vi "Main RT 2.vi"() -> ()   [LabVIEW 2015]
uses:
  <vilib>/RioEmbeddedCAN/RioEmbeddedCAN.llb/CANFrameControl.ctl
  Enum nastawy 2.ctl
  <vilib>/Platform/TimedLoop/XDataNode/timing_clust.ctl
  <vilib>/Platform/TimedLoop/XDataNode/nitl_modes.ctl
  <vilib>/Platform/TimedLoop/XDataNode/wakeup.ctl
  <vilib>/FPGAPlugInAG/sbRIO-9636/niLvFpga_Open_sbRIO-9636.vi
  <vilib>/rvi/interface/common/dynamic/niFpgaDynamicAddResources.vi
  <vilib>/FPGAPlugInAG/Dynamic/niLvFpga_Reset_Dynamic.vi
  <vilib>/FPGAPlugInAG/Dynamic/niLvFpga_Run_Dynamic.vi
  <vilib>/FPGAPlugInAG/Dynamic/niLvFpga_Close_Dynamic.vi
  <vilib>/platform/TimedLoop/XDataNode/XDataNode.xnode
  <vilib>/rvi/interface/nirviOpenFPGA/nirviOpenFPGA.xnode
  FPGA Bitfiles/Raptorv2_FPGATarget_FPGAMain_nw1CBh-YlYM.lvbitx
  FPGA/Main FPGA.vi
  <vilib>/rvi/interface/nirviMethod/nirviMethod.xnode
  <vilib>/rvi/interface/nirviCloseFPGA/nirviCloseFPGA.xnode
  <vilib>/Platform/TimedLoop/XDataNode/XDNodeRunTimeDep.lvlib
  <vilib>/robotics/Protocols/NMEA/NMEA API.lvlib
  <vilib>/Instr/_visa.llb/VISA Configure Serial Port (Instr).vi
  <resource>/objmgr/RioEmbeddedCANInterface.rc
panel:
  out "specific error cleared?":bool
  in  "Boolean":bool
  in  "ramki jazdy 2":T1[](array[typedef]) {"type" items=["CAN Data", "CAN Remote"]; "identifier" format="%.0x"}
  out "Numeric":i32
  out "# pending insert":i32
  out "# pending remove":i32
  out "# elements in queue":i32
  out "current time":timestamp
  out "Delay":dbl
  out "Odebrane wiadomości z PC":dbl
  out "CAN frame":T1 {"type" items=["CAN Data", "CAN Remote"]; "identifier" format="%.0x"}
  out "Przestarzała data":bool caption="Time has Elapsed"
  out "longitude (deg) 2":dbl format="%#_8g"
  out "latitude (deg) 2":dbl format="%#_8g"
  in  "VISA resource name":refnum<visa-resource-name>="ASRL1::INSTR"
  out "longitude (deg)":i64
  out "latitude (deg)":i64
  out "GPS data":T2 {"oldest read timestamp" format="%^<%.3X\n%x>T"; "latitude (deg)" format="%#_10g"; "longitude (deg)" format="%#_10g"}
  out "wyczyszczona":bool=TRUE
  in  "Wyczyśćkolejke":bool
  in  "stop wysylanie":bool
  in  "odczyt CAN-a":bool=TRUE
  out "ilosc mesagy READ CAN":dbl
  in  "Pokaz odczytany CAN":bool=TRUE
  out "CAN Frames":string[][](table) caption="Frames"
  in  "stop odczyt can":bool
  in  "Hexadecimal?":bool
  in  "stop zapis can":bool
  out "new data":bool
  out "ramki jazdy":T1[](array[typedef]) {"type" items=["CAN Data", "CAN Remote"]; "identifier" format="%.0x"}
  in  "odbior udp":bool
  out "ramki konf":T1 {"type" items=["CAN Data", "CAN Remote"]; "identifier" format="%.0x"}
  in  "Number of Frames to Display":i32=5
  in  "receive queue size":u32=500
  in  "baud rate":u32=500000
  in  "interface index":u32
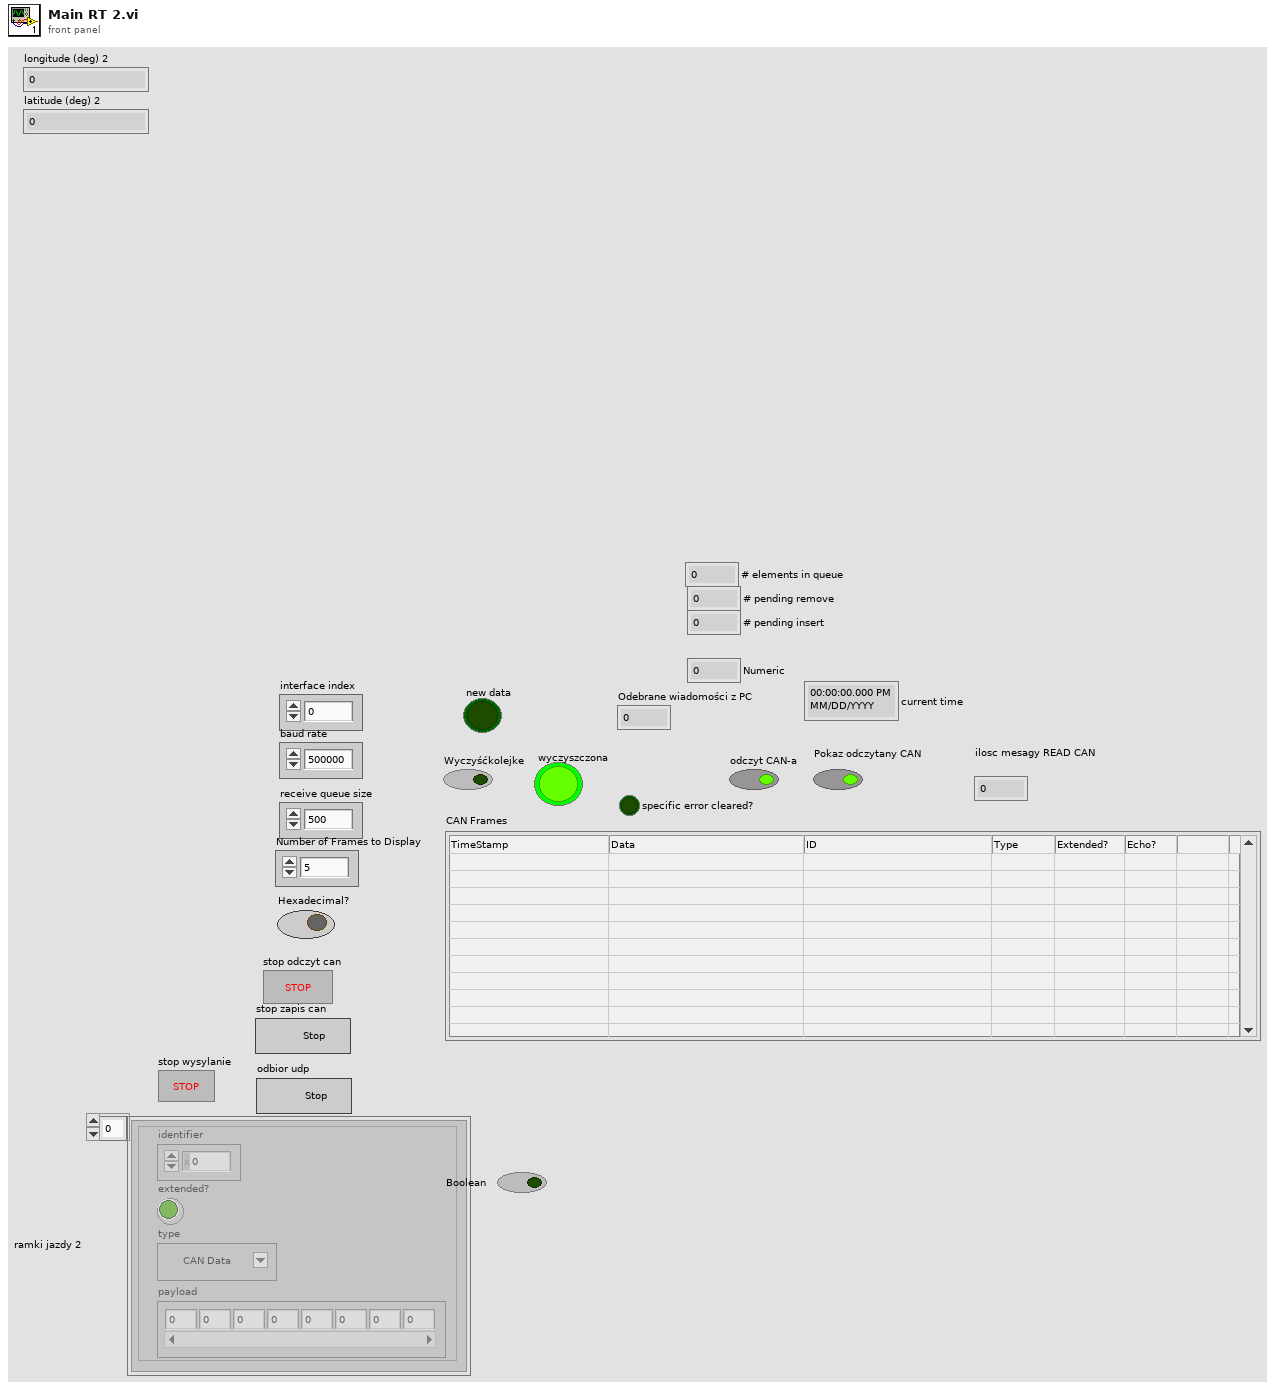
[diagram p1: front panel]
types:
  T1 = typedef "CANFrameControl.ctl" = cluster{"identifier":u32, "extended?":bool, "type":u8, "payload":u8[]}
  T2 = cluster{"oldest read timestamp":timestamp, "latitude (deg)":dbl, "longitude (deg)":dbl, "ground speed (knots)":dbl, "true track angle (deg)":dbl, "altitude above mean sea level (m)":dbl}
  T3 = typedef "Enum nastawy 2.ctl" = enum16{"STOP", "PRZOD P", "SRODEK P", "TYL P", "PRZOD L", "SRODEK L", "TYL L"}
  T4 = typedef "XDNodeRunTimeDep.lvlib/timing_clust.ctl" = cluster{"Expected End [f-1]":u64, "Actual End [f-1]":u64, "Finished Late? [f-1]":bool, "Expected End [i-1]":u64, "Actual End [i-1]":u64, "Finished Late? [i-1]":bool, "Expected Start [i]":u64, "Actual Start [i]":u64, "Expected Start [f]":u64, "Actual Start [f]":u64, "Source Name":string, "Structure Name":string, "Period":i64, "Deadline":i64, "Offset":i64, "Start":i64, "Priority":i32, "Timeout":i32, "Mode":T5, "Wakeup Reason":T6, "Error":errorcluster, "Source Type":string, "Secondary Source Type":string, "Global End Time":u64, "Global Start Time":u64, "Frame Duration":u64, "Iteration Duration":u64, "Assigned CPU":i32, "I/O Scan Engine Mode":u32}
  T5 = typedef "XDNodeRunTimeDep.lvlib/nitl_modes.ctl" = enum32{"No Change", "Process missed periods, maintain original phase", "Discard missed periods, maintain original phase", "Process missed periods, ignore original phase", "Discard missed periods, ignore original phase"}
  T6 = typedef "XDNodeRunTimeDep.lvlib/wakeup.ctl" = enum32{"Normal", "Aborted", "Asynchronous wakeup", "Timing source error", "Timed loop error", "Timeout"}
  T7 = cluster{"type":string, "Cluster":cluster{"date/time string":string, "array of cans":T1[]}, "bool":bool}
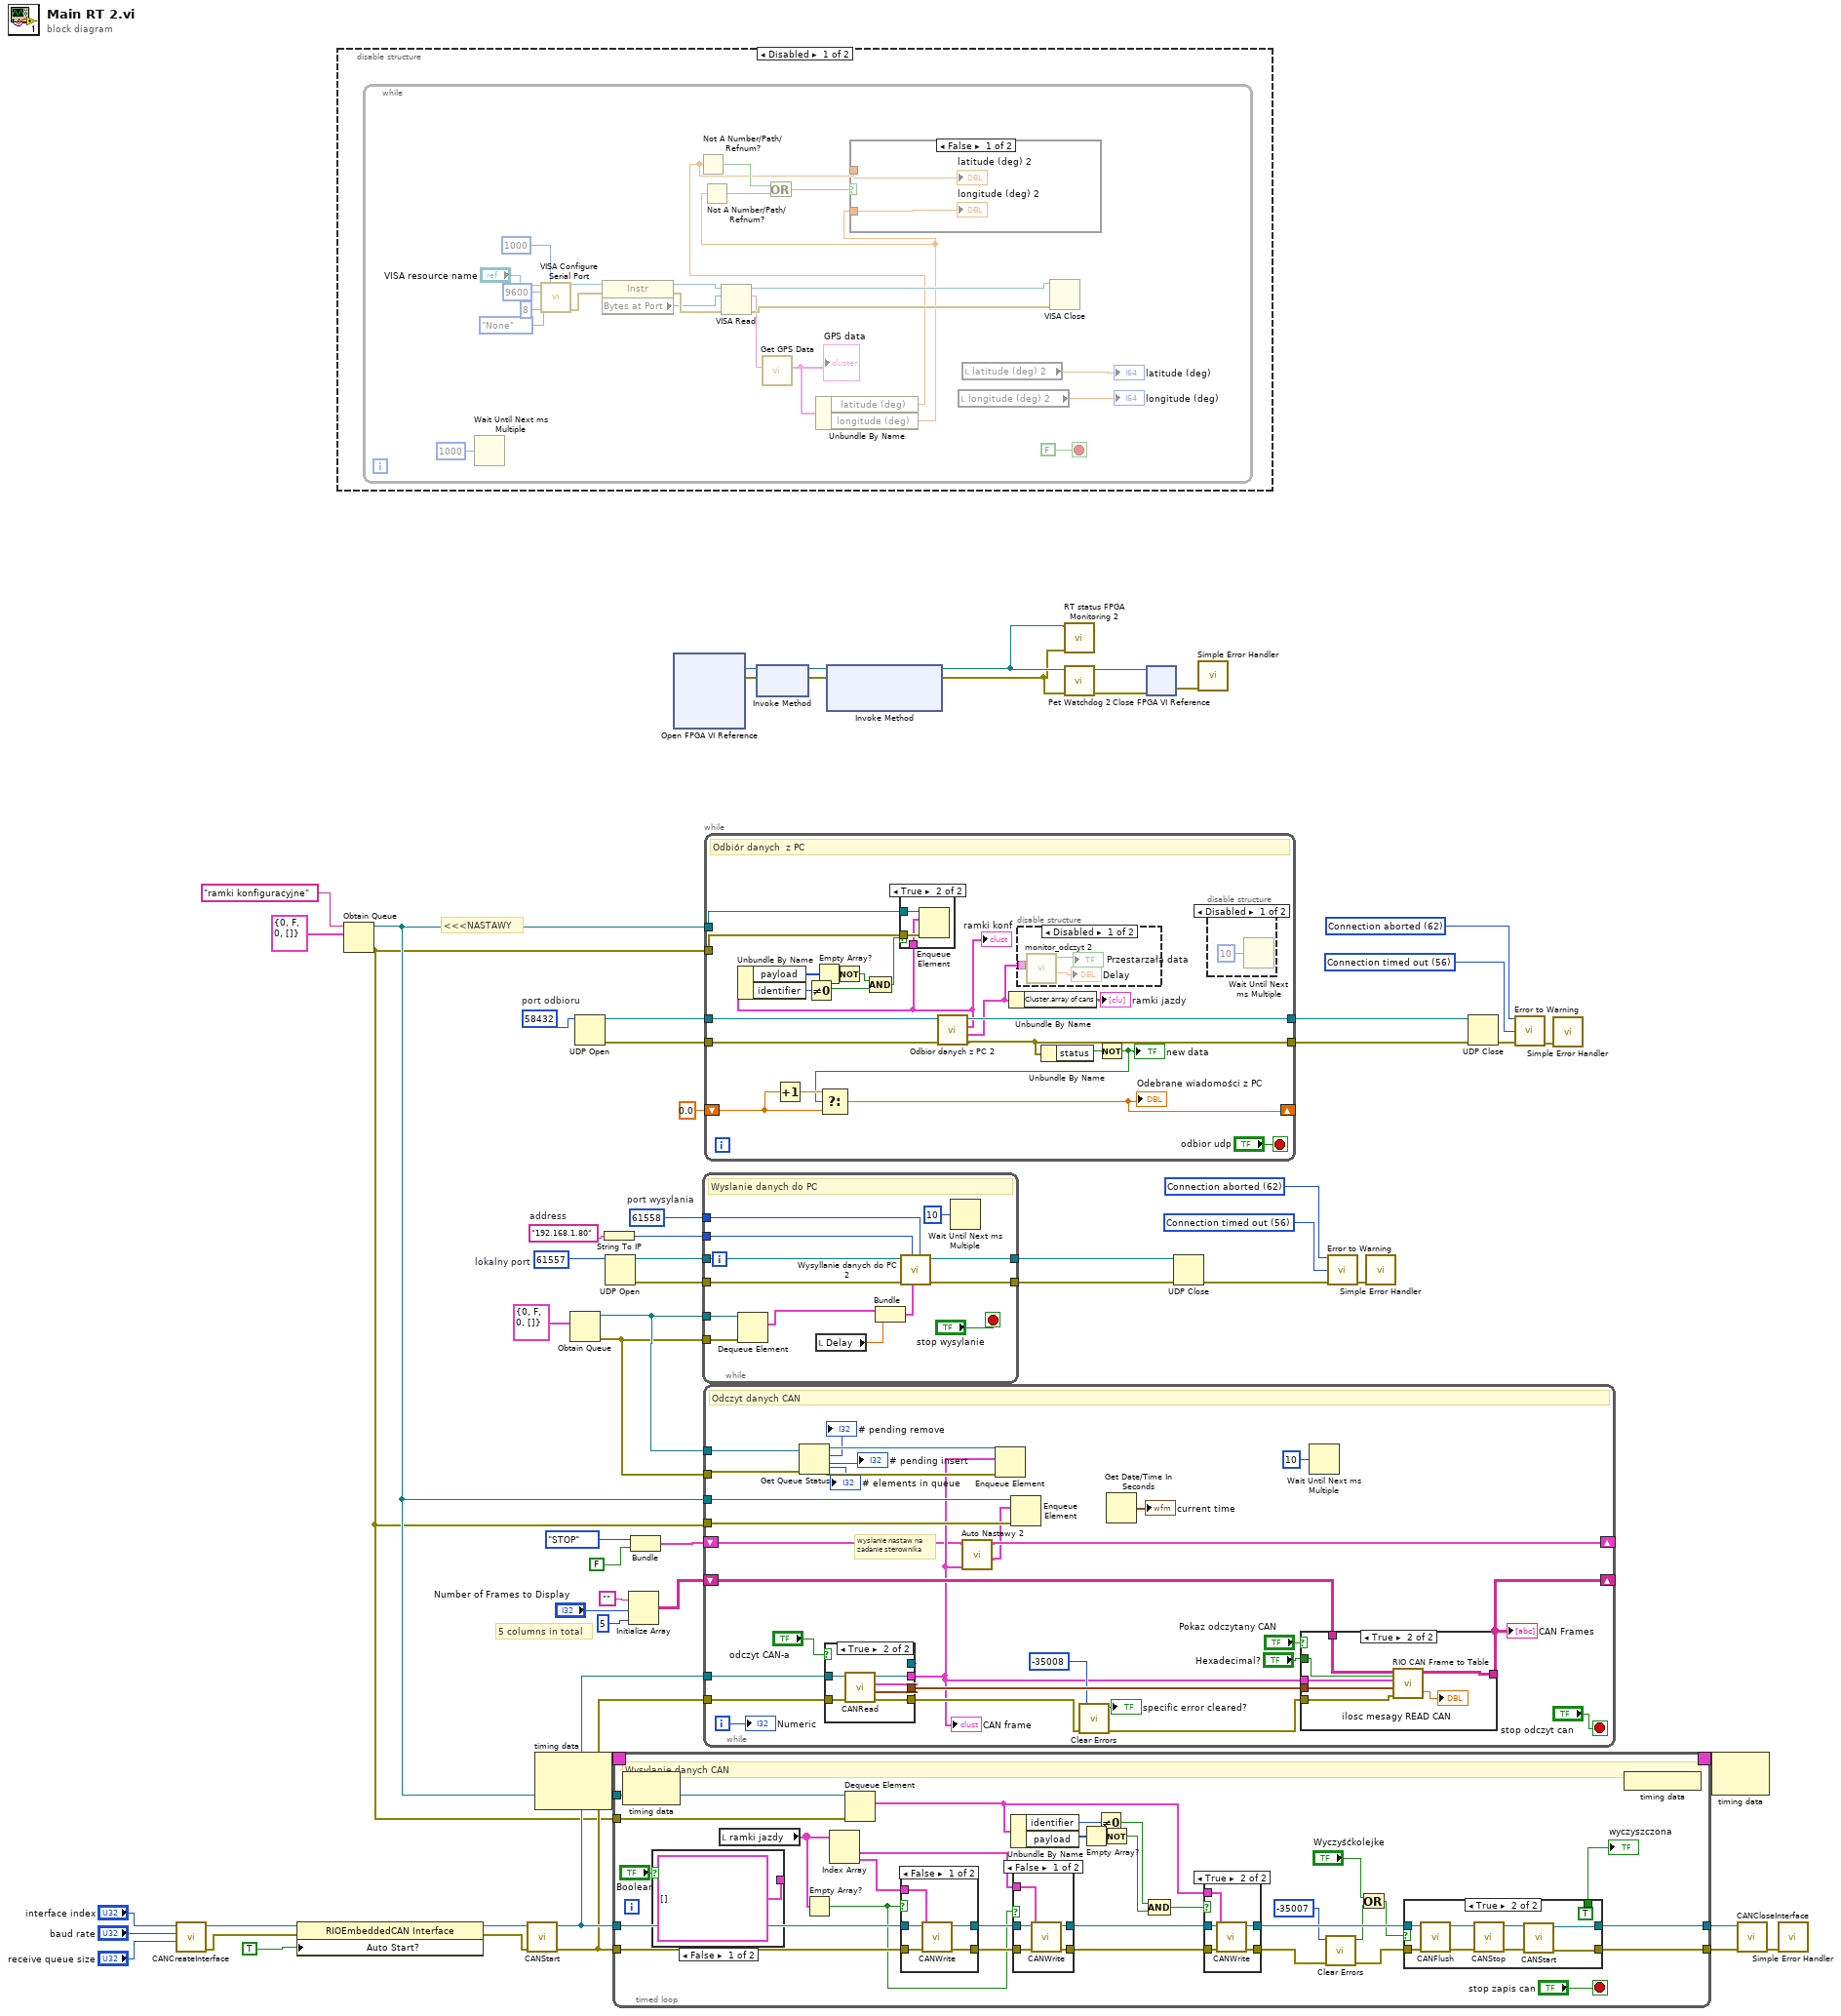
[diagram p0: block diagram]
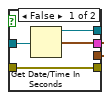
[diagram p3: hidden frame]
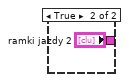
[diagram p9: hidden frame]
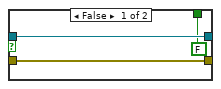
[diagram p10: hidden frame]
diagram:
  w22 = u16 58432  # port odbioru
  w26 = 56 items=["No Error", "Argument Error", "Memory Full", "Out of Zone", "End of File", "File Already Open", "Generic File IO Error", "File Not Found", "File Permission Error", "Disk Full", "Duplicate Path", "Too Many Files Open", "Not Enabled", "Resource File Not Found", "Cannot Add Resource", "Resource Not Found", "Image Not Found", "Image Memory Error", "Pen Does Not Exist", "Config Bad Type", "Config Token Not Found", "Config Parse Error", "Config Memory Error", "Bad External Code Format", "Bad External Code Offset", "External Code Not Present", "Null Window", "Destroy Window Mixup", "Null Menu", "Print Aborted", "Bad Print Record", "Print Driver Error", "Windows Error During Print", "Memory Error During Print", "Print Dialog Error", "Generic Print Error", "Invalid Device Refnum", "Device Not Found", "Device Parameter Error", "Device Unit Error", "Can't Open Device", "Device Call Aborted", "Generic Error", "Cancelled By User", "Object ID Too Low", "Object ID Too High", "Object Not In Heap", "Unknown Heap", "Bad DefProc ID", "DefProc Not In Table", "Message Out Of Range", "Null Method", "Unknown Message", "Manager Call Not Supported", "Bad address", "Connection In progress", "Connection timed out", "Connection is already in progress", "Network attribute not supported", "Network error", "Address in use", "System out of memory", "Connection aborted", "Connection refused", "Connection is not connected", "Connection is already connected", "Connection closed", "Initialize error (interapplication manager)", "Bad occurrence", "Wait on unbound occurrence handler", "Occurrence queue overflow", "Bad path", "Semaphore not signaled", "Unrecognized type (interapplication manager)"] ("3rd Error to Convert")
  w25 = 62 items=["No Error", "Argument Error", "Memory Full", "Out of Zone", "End of File", "File Already Open", "Generic File IO Error", "File Not Found", "File Permission Error", "Disk Full", "Duplicate Path", "Too Many Files Open", "Not Enabled", "Resource File Not Found", "Cannot Add Resource", "Resource Not Found", "Image Not Found", "Image Memory Error", "Pen Does Not Exist", "Config Bad Type", "Config Token Not Found", "Config Parse Error", "Config Memory Error", "Bad External Code Format", "Bad External Code Offset", "External Code Not Present", "Null Window", "Destroy Window Mixup", "Null Menu", "Print Aborted", "Bad Print Record", "Print Driver Error", "Windows Error During Print", "Memory Error During Print", "Print Dialog Error", "Generic Print Error", "Invalid Device Refnum", "Device Not Found", "Device Parameter Error", "Device Unit Error", "Can't Open Device", "Device Call Aborted", "Generic Error", "Cancelled By User", "Object ID Too Low", "Object ID Too High", "Object Not In Heap", "Unknown Heap", "Bad DefProc ID", "DefProc Not In Table", "Message Out Of Range", "Null Method", "Unknown Message", "Manager Call Not Supported", "Bad address", "Connection In progress", "Connection timed out", "Connection is already in progress", "Network attribute not supported", "Network error", "Address in use", "System out of memory", "Connection aborted", "Connection refused", "Connection is not connected", "Connection is already connected", "Connection closed", "Initialize error (interapplication manager)", "Bad occurrence", "Wait on unbound occurrence handler", "Occurrence queue overflow", "Bad path", "Semaphore not signaled", "Unrecognized type (interapplication manager)"] ("1st Error to Convert")
  w35 = u16 61557  # lokalny port
  w33 = u16 61558  # port wysylania
  w34 = "192.168.1.80"  # address
  w37 = 56 items=["No Error", "Argument Error", "Memory Full", "Out of Zone", "End of File", "File Already Open", "Generic File IO Error", "File Not Found", "File Permission Error", "Disk Full", "Duplicate Path", "Too Many Files Open", "Not Enabled", "Resource File Not Found", "Cannot Add Resource", "Resource Not Found", "Image Not Found", "Image Memory Error", "Pen Does Not Exist", "Config Bad Type", "Config Token Not Found", "Config Parse Error", "Config Memory Error", "Bad External Code Format", "Bad External Code Offset", "External Code Not Present", "Null Window", "Destroy Window Mixup", "Null Menu", "Print Aborted", "Bad Print Record", "Print Driver Error", "Windows Error During Print", "Memory Error During Print", "Print Dialog Error", "Generic Print Error", "Invalid Device Refnum", "Device Not Found", "Device Parameter Error", "Device Unit Error", "Can't Open Device", "Device Call Aborted", "Generic Error", "Cancelled By User", "Object ID Too Low", "Object ID Too High", "Object Not In Heap", "Unknown Heap", "Bad DefProc ID", "DefProc Not In Table", "Message Out Of Range", "Null Method", "Unknown Message", "Manager Call Not Supported", "Bad address", "Connection In progress", "Connection timed out", "Connection is already in progress", "Network attribute not supported", "Network error", "Address in use", "System out of memory", "Connection aborted", "Connection refused", "Connection is not connected", "Connection is already connected", "Connection closed", "Initialize error (interapplication manager)", "Bad occurrence", "Wait on unbound occurrence handler", "Occurrence queue overflow", "Bad path", "Semaphore not signaled", "Unrecognized type (interapplication manager)"] ("3rd Error to Convert")
  w18 = 62 items=["No Error", "Argument Error", "Memory Full", "Out of Zone", "End of File", "File Already Open", "Generic File IO Error", "File Not Found", "File Permission Error", "Disk Full", "Duplicate Path", "Too Many Files Open", "Not Enabled", "Resource File Not Found", "Cannot Add Resource", "Resource Not Found", "Image Not Found", "Image Memory Error", "Pen Does Not Exist", "Config Bad Type", "Config Token Not Found", "Config Parse Error", "Config Memory Error", "Bad External Code Format", "Bad External Code Offset", "External Code Not Present", "Null Window", "Destroy Window Mixup", "Null Menu", "Print Aborted", "Bad Print Record", "Print Driver Error", "Windows Error During Print", "Memory Error During Print", "Print Dialog Error", "Generic Print Error", "Invalid Device Refnum", "Device Not Found", "Device Parameter Error", "Device Unit Error", "Can't Open Device", "Device Call Aborted", "Generic Error", "Cancelled By User", "Object ID Too Low", "Object ID Too High", "Object Not In Heap", "Unknown Heap", "Bad DefProc ID", "DefProc Not In Table", "Message Out Of Range", "Null Method", "Unknown Message", "Manager Call Not Supported", "Bad address", "Connection In progress", "Connection timed out", "Connection is already in progress", "Network attribute not supported", "Network error", "Address in use", "System out of memory", "Connection aborted", "Connection refused", "Connection is not connected", "Connection is already connected", "Connection closed", "Initialize error (interapplication manager)", "Bad occurrence", "Wait on unbound occurrence handler", "Occurrence queue overflow", "Bad path", "Semaphore not signaled", "Unrecognized type (interapplication manager)"] ("1st Error to Convert")
  # "<<<NASTAWY"
  # "5 columns in total"
  n1 = call <vilib>:"CANCreateInterface.vi"("receive queue size (5)"="receive queue size", "baud rate (125000 bps)"="baud rate", "interface index"="interface index") -> ("error out"=w7:errorcluster, "interface object out"=w10:refnum<k20>)  [unwired: 7 in]
  n2 = property class="RIOEmbeddedCAN Interface"(reference=w10, error in=w7, "Auto Start?"=TRUE) -> (reference out=w8:refnum<k20>, error out=w6:errorcluster)
  n3 = disable-structure shown="Disabled" {
    frame Disabled {
      n4 = while {
        stop <- FALSE stop-if-true
        n5 = Wait Until Next ms Multiple(millisecond multiple=u32 1000) -> ()  [unwired: 1 out]
        n6 = call-poly "VISA Configure Serial Port"("VISA resource name"="VISA resource name", "timeout (10sec)"=u32 1000, "baud rate (9600)"=u32 9600, "data bits (8)"=u16 8, "parity (0:none)"=enum16{"None", "Odd", "Even", "Mark", "Space"}."None") -> ("VISA resource name out"=w80:refnum<visa-resource-name>, "error out"=w79:errorcluster)  [unwired: 9 in]
        n7 = property class="Instr"(reference=w80, error in=w79) -> (reference out=w81:refnum<visa-resource-name>, error out=w78:errorcluster, "Bytes at Port"=w74:u32)
        n8 = VISA Read(VISA resource name=w81, byte count=w74, error in (no error)=w78) -> (VISA resource name out=w82:refnum<visa-resource-name>, read buffer=w76:string, error out=w77:errorcluster)  [unwired: 1 out]
        n9 = call <vilib>:"Get GPS Data.vi"("sensor data"=w76) -> ("GPS data"=w75:T2)  [unwired: 8 in, 2 out]
        "GPS data" <- w75
        n10 = Unbundle By Name(w75) -> ("latitude (deg)"=w64:dbl, "longitude (deg)"=w62:dbl)
        n11 = Not A Number/Path/Refnum?(number/path/refnum=w64) -> (NaN/Path/Refnum?=w67:bool)
        n12 = Not A Number/Path/Refnum?(number/path/refnum=w62) -> (NaN/Path/Refnum?=w66:bool)
        n13 = Or(x=w67, y=w66) -> (x .or. y?=w65:bool)
        n14 = case shown="False" w65 {
          tunnel: w62 -> [w85 _]
          tunnel: w64 -> [w84 _]
          frame False {
            "longitude (deg) 2" <- w85
            "latitude (deg) 2" <- w84
          }
          frame True {
          }
        }
        n15 = local read "longitude (deg) 2"() -> (→"longitude (deg)":dbl)
        n16 = local read "latitude (deg) 2"() -> (→"latitude (deg)":dbl)
        n17 = VISA Close(VISA resource name=w82, error in (no error)=w77) -> ()  [unwired: 1 out]
      }
    }
    frame Enabled {
    }
  }
  n18 = Obtain Queue(name (unnamed)="ramki konfiguracyjne", element data type=T1 {"identifier"=0, "extended?"=FALSE, "type"=0, "payload"=[]} ("ramki konf")) -> (queue out=w15:refnum<queue>, error out=w14:errorcluster)  [unwired: 3 in, 1 out]
  n19 = call <vilib>:"CANStart.vi"("error in (no error)"=w6, "interface object in"=w8) -> ("error out"=w47:errorcluster, "interface object out"=w48:refnum<k20>)  [unwired: 8 in]
  n20 = node-c288() -> (w60:T4)  [unwired: 2 in]
  n21 = Obtain Queue(element data type=T1 {"identifier"=0, "extended?"=FALSE, "type"=0, "payload"=[]} ("CAN frame")) -> (queue out=w12:refnum<queue>, error out=w11:errorcluster)  [unwired: 4 in, 1 out]
  n22 = UDP Open(11:w22) -> (port=w39:refnum<k16>, 0:w40:errorcluster)  [unwired: 4 in, 1 out]
  n23 = String To IP(1:w34) -> (0:w32:u32)
  n24 = UDP Open(11:w35) -> (port=w31:refnum<k16>, 0:w30:errorcluster)  [unwired: 4 in, 1 out]
  n25 = timed-loop "Timed Loop" {
    tunnel: w48 -> [w103]
    tunnel: w47 -> [w102]
    tunnel: [w101] -> w51
    tunnel: [w100] -> w50
    timing: w60 -> [_]
    timing-out: [_] -> w59
    tunnel: w15 -> [w91]
    tunnel: w14 -> [w90]
    stop <- "stop zapis can" stop-if-true
    # "Wysylanie danych CAN"
    n26 = node-c288() -> ()  [unwired: 1 in, 1 out]
    n27 = case shown="False" "Boolean" {
      tunnel: [T1[] [] ("ramki jazdy 2") "ramki jazdy 2"] -> _
      frame False {
      }
      frame True {
      }
    }
    n28 = local read "ramki jazdy"() -> (w86:T1[])
    n29 = Empty Array?(array=w86) -> (empty?=w88:bool)
    n30 = Index Array(array=w86) -> (element #1=w114:T1, element #2=w113:T1)  [unwired: 2 in]
    n31 = Dequeue Element(queue=w91, error in (no error)=w90) -> (element=w89:T1)  [unwired: 1 in, 3 out]
    n32 = case shown="False" w88 {
      tunnel: w103 -> [w151 w152]
      tunnel: w102 -> [w150 w153]
      tunnel: [w148 w152] -> w115
      tunnel: [w147 w153] -> w116
      tunnel: w113 -> [w149 _]
      frame False {
        n33 = call <vilib>:"CANWrite.vi"("error in (no error)"=w150, "CAN frame"=w149, "interface object in"=w151) -> ("error out"=w147:errorcluster, "interface object out"=w148:refnum<k20>)  [unwired: 7 in]
      }
      frame True {
      }
    }
    n34 = Unbundle By Name(w89) -> ("identifier"=w109:u32, "payload"=w110:u8[])
    n35 = case shown="False" w88 {
      tunnel: w116 -> [w144 w146]
      tunnel: [w142 w145] -> w112
      tunnel: [w141 w146] -> w111
      tunnel: w115 -> [w143 w145]
      tunnel: w114 -> [w140 _]
      frame False {
        n36 = call <vilib>:"CANWrite.vi"("error in (no error)"=w144, "CAN frame"=w140, "interface object in"=w143) -> ("error out"=w141:errorcluster, "interface object out"=w142:refnum<k20>)  [unwired: 7 in]
      }
      frame True {
      }
    }
    n37 = Empty Array?(array=w110) -> (empty?=w106:bool)
    n38 = Not Equal To 0?(x=w109) -> (x != 0?=w107:bool)
    n39 = Not(x=w106) -> (.not. x?=w105:bool)
    n40 = Compound Arithmetic op=AND(w107, w105) -> (w108:bool)
    n41 = case shown="True" w108 {
      tunnel: w111 -> [w132 w137]
      tunnel: [w131 w134] -> w99
      tunnel: [w132 w133] -> w104
      tunnel: w112 -> [w131 w136]
      tunnel: w89 -> [_ w135]
      frame False {
      }
      frame True {
        n42 = call <vilib>:"CANWrite.vi"("error in (no error)"=w137, "CAN frame"=w135, "interface object in"=w136) -> ("error out"=w133:errorcluster, "interface object out"=w134:refnum<k20>)  [unwired: 7 in]
      }
    }
    n43 = call <vilib>:"Clear Errors.vi"("error in (no error)"=w104, "specific error code to clear (0: all)"=-35007) -> ("error out"=w96:errorcluster, "specific error cleared?"=w94:bool)  [unwired: 4 in]
    n44 = Or(x="Wyczyśćkolejke", y=w94) -> (x .or. y?=w95:bool)
    n45 = case shown="True" w95 {
      tunnel: [w121 w123] -> w101
      tunnel: [w120 w122] -> w100
      tunnel: w99 -> [w121 w130]
      tunnel: w96 -> [w120 w129]
      tunnel: [FALSE TRUE] -> w92
      frame False {
      }
      frame True {
        n46 = call <vilib>:"CANFlush.vi"("error in (no error)"=w129, "interface object in"=w130) -> ("error out"=w126:errorcluster, "interface object out"=w127:refnum<k20>)  [unwired: 8 in]
        n47 = call <vilib>:"CANStop.vi"("error in (no error)"=w126, "interface object in"=w127) -> ("error out"=w125:errorcluster, "interface object out"=w124:refnum<k20>)  [unwired: 8 in]
        n48 = call <vilib>:"CANStart.vi"("error in (no error)"=w125, "interface object in"=w124) -> ("error out"=w122:errorcluster, "interface object out"=w123:refnum<k20>)  [unwired: 8 in]
      }
    }
    "wyczyszczona" <- w92
    n49 = node-c288() -> ()  [unwired: 1 out]
  }
  n50 = Initialize Array("" ("Empty String Constant"), "Number of Frames to Display", 5 ("dimension size")) -> (w49:string[][])
  n51 = Bundle("Enum"=Enum_nastawy_2."STOP", FALSE) -> (w17:cluster{"Enum":T3, bool})  [unwired: 1 in]
  n52 = xnode "Open FPGA VI Reference"() -> ("FPGA VI Reference Out"=w43:refnum<k20>, "error out"=w44:errorcluster)  [unwired: 2 in]
  n53 = while {
    tunnel: w33 -> [w158]
    tunnel: w32 -> [w159]
    tunnel: w31 -> [w160]
    tunnel: w30 -> [w155]
    tunnel: [w157] -> w29
    tunnel: [w156] -> w28
    tunnel: w12 -> [w163]
    tunnel: w11 -> [w162]
    stop <- "stop wysylanie" stop-if-true
    # "Wyslanie danych do PC"
    n54 = Dequeue Element(queue=w163, error in (no error)=w162) -> (element=w161:T1)  [unwired: 1 in, 3 out]
    n55 = local read "Delay"() -> (w164:dbl)
    n56 = Bundle("CAN frame"=w161, "Delay"=w164) -> (w154:cluster{"CAN frame":T1, "Delay":dbl})  [unwired: 1 in]
    n57 = call "Wysyllanie danych do PC  2.vi"("remote port"=w158, "output cluster"=w154, "adres"=w159, "error in (no error)"=w155, "UDP Network Connection in"=w160) -> ("error out"=w156:errorcluster, "UDP Network Connection out"=w157:refnum<k16>)  [unwired: 5 in]
    n58 = Wait Until Next ms Multiple(millisecond multiple=u32 10) -> ()  [unwired: 1 out]
  }
  n59 = while "Timed Loop" {
    shift-right: [w188] -> _
    shift-left: w49 -> [w189]
    tunnel: w48 -> [w195]
    tunnel: w47 -> [w194]
    shift-right: [w168] -> _
    shift-left: w17 -> [w169]
    tunnel: w15 -> [w193]
    tunnel: w14 -> [w192]
    tunnel: w12 -> [w191]
    tunnel: w11 -> [w190]
    i -> [w177]
    stop <- "stop odczyt can" stop-if-true
    # "wyslanie nastaw na \nzadanie sterownika"
    # "Odczyt danych CAN"
    n60 = Get Queue Status(queue=w191, error in (no error)=w190) -> (queue out=w182:refnum<queue>, # pending remove=→"# pending remove":i32, # pending insert=→"# pending insert":i32, error out=w181:errorcluster, # elements in queue=→"# elements in queue":i32)  [unwired: 1 in, 3 out]
    n61 = case shown="True" "odczyt CAN-a" {
      tunnel: w195 -> [w205 w212]
      tunnel: w194 -> [w206 w211]
      tunnel: [w204 w210] -> w186
      tunnel: [w206 w209] -> w174
      tunnel: [_ w207] -> w170
      tunnel: [w205 w208] -> _
      frame False {
        n62 = Get Date/Time In Seconds() -> (seconds since 1Jan1904=w204:timestamp)
      }
      frame True {
        n63 = call <vilib>:"CANRead.vi"("error in (no error)"=w211, "interface object in"=w212) -> ("error out"=w209:errorcluster, "timestamp"=w210:timestamp, "CAN frame"=w207:T1, "interface object out"=w208:refnum<k20>)  [unwired: 6 in]
      }
    }
    "CAN frame" <- w170
    n64 = call "Auto Nastawy 2.vi"("CAN ramki in"=w170, "Auto N in"=w169) -> ("CAN konifguracyjny"=w167:T1, "Auto N out"=w168:cluster{"Enum":T3, bool})  [unwired: 8 in]
    n65 = Enqueue Element(queue=w182, element=w170, error in (no error)=w181) -> ()  [unwired: 1 in, 3 out]
    n66 = Enqueue Element(queue=w193, element=w167, error in (no error)=w192) -> ()  [unwired: 1 in, 3 out]
    n67 = call <vilib>:"Clear Errors.vi"("error in (no error)"=w174, "specific error code to clear (0: all)"=-35008) -> ("error out"=w173:errorcluster, "specific error cleared?"=→"specific error cleared?":bool)  [unwired: 4 in]
    n68 = Get Date/Time In Seconds() -> (seconds since 1Jan1904=→"current time":timestamp)
    n69 = case shown="True" "Pokaz odczytany CAN" {
      tunnel: [w196 w203] -> w188
      tunnel: w189 -> [w196 w201]
      tunnel: w186 -> [_ w200]
      tunnel: w170 -> [_ w199]
      tunnel: w173 -> [_ w198]
      tunnel: "Hexadecimal?" -> [_ w197]
      frame False {
      }
      frame True {
        n70 = call "RIO CAN Frame to Table.vi"("Hexadecimal?"=w197, "error in (no error)"=w198, "timestamp"=w200, "CAN frame"=w199, "Old CAN Frames"=w201) -> ("New CAN Frames"=w203:string[][], "Ilość wiadomości CAN odebranych"=→"ilosc mesagy READ CAN":dbl)  [unwired: 5 in]
      }
    }
    "CAN Frames" <- w188
    n71 = Wait Until Next ms Multiple(millisecond multiple=u32 10) -> ()  [unwired: 1 out]
    "Numeric" <- w177
  }
  n72 = while {
    tunnel: w39 -> [w218]
    tunnel: w40 -> [w217]
    tunnel: [w216] -> w41
    tunnel: [w215] -> w23
    tunnel: w15 -> [w231]
    tunnel: w14 -> [w230]
    shift-right: [w223] -> _
    shift-left: 0.0 -> [w222]
    stop <- "odbior udp" stop-if-true
    # "Odbiór danych  z PC"
    n73 = Increment(x=w222) -> (x+1=w224:dbl)
    n74 = call "Odbior danych z PC 2.vi"("error in (no error)"=w217, "connection ID"=w218) -> ("error out"=w216:errorcluster, "output cluster"=w213:T7, "konf"=w214:T1, "connection ID out"=w215:refnum<k16>)  [unwired: 6 in]
    "ramki konf" <- w214
    n75 = Unbundle By Name(w214) -> ("payload"=w228:u8[], "identifier"=w229:u32)
    n76 = Not Equal To 0?(x=w229) -> (x != 0?=w226:bool)
    n77 = Empty Array?(array=w228) -> (empty?=w220:bool)
    n78 = Not(x=w220) -> (.not. x?=w227:bool)
    n79 = Compound Arithmetic op=AND(w227, w226) -> (w225:bool)
    n80 = case shown="True" w225 {
      tunnel: w231 -> [_ w239]
      tunnel: w230 -> [_ w238]
      tunnel: w214 -> [_ w237]
      frame False {
      }
      frame True {
        n81 = Enqueue Element(queue=w239, element=w237, error in (no error)=w238) -> ()  [unwired: 1 in, 3 out]
      }
    }
    n82 = Unbundle By Name(w213) -> ("Cluster.array of cans"=→"ramki jazdy":T1[])
    n83 = disable-structure shown="Disabled" {
      disable-tunnel: w213 -> [w234 _]
      frame Disabled {
        n84 = call "monitor_odczyt 2.vi"("output cluster"=w234) -> ("Delay"=→"Delay":dbl, "Przestarzała data"=→"Przestarzała data":bool)  [unwired: 8 in, 1 out]
      }
      frame Enabled {
      }
    }
    n85 = Unbundle By Name(w216) -> ("status"=w232:bool)
    n86 = Not(x=w232) -> (.not. x?=w221:bool)
    "new data" <- w221
    n87 = Select(t=w224, s=w221, f=w222) -> (s? t:f=w223:dbl)
    "Odebrane wiadomości z PC" <- w223
    n88 = disable-structure shown="Disabled" {
      frame Disabled {
        n89 = Wait Until Next ms Multiple(millisecond multiple=u32 10) -> ()  [unwired: 1 out]
      }
      frame Enabled {
      }
    }
  }
  n90 = xnode "Invoke Method"("FPGA VI Reference In"=w43, "error in"=w44) -> ("FPGA VI Reference Out"=w45:refnum<k20>, "error out"=w46:errorcluster)
  n91 = xnode "Invoke Method"("FPGA VI Reference In"=w45, "error in"=w46) -> ("FPGA VI Reference Out"=w4:refnum<k20>, "error out"=w1:errorcluster)  [unwired: 1 in]
  n92 = call "RT status FPGA Monitoring 2.vi"("error in (no error)"=w1, "FPGA VI Reference Out 2"=w4) -> ()  [unwired: 10 in]
  n93 = call "Pet Watchdog 2.vi"("error in (no error)"=w1, "FPGA VI Reference Out"=w4) -> ("error out"=w2:errorcluster, "FPGA VI Reference Out 2"=w3:refnum<k20>)  [unwired: 8 in]
  n94 = xnode "Close FPGA VI Reference"("FPGA VI Reference In"=w3, "error in"=w2) -> ("error out"=w42:errorcluster)
  n95 = UDP Close(connection ID=w29, 8:w28) -> (error out=w38:errorcluster)  [unwired: 1 out]
  n96 = call <vilib>:"Simple Error Handler.vi"("error in (no error)"=w42) -> ()  [unwired: 1 in, 8 out]
  n97 = call <vilib>:"Error to Warning.vi"("1st Error to Convert"=w18, "3rd Error to Convert"=w37, "error in"=w38) -> ("warning out"=w36:errorcluster)  [unwired: 3 in, 9 out]
  n98 = call <vilib>:"Simple Error Handler.vi"("error in (no error)"=w36) -> ()  [unwired: 1 in, 8 out]
  n99 = UDP Close(connection ID=w23, 8:w41) -> (error out=w24:errorcluster)  [unwired: 1 out]
  n100 = call <vilib>:"Error to Warning.vi"("1st Error to Convert"=w25, "3rd Error to Convert"=w26, "error in"=w24) -> ("warning out"=w27:errorcluster)  [unwired: 3 in, 9 out]
  n101 = call <vilib>:"Simple Error Handler.vi"("error in (no error)"=w27) -> ()  [unwired: 1 in, 8 out]
  n102 = node-c288(w59) -> ()  [unwired: 1 out]
  n103 = call <vilib>:"CANCloseInterface.vi"("error in (no error)"=w50, "interface object in"=w51) -> ("error out"=w52:errorcluster)  [unwired: 9 in]
  n104 = call <vilib>:"Simple Error Handler.vi"("error in (no error)"=w52) -> ()  [unwired: 4 in, 5 out]
